vi "Init.vi"(8 "error in (no error)":errorcluster, 11 "RT_Sprite in":refnum<class "RT_Sprite.lvclass">) -> (0 "error out":errorcluster, 3 "RT_Sprite out":refnum<class "RT_Sprite.lvclass">)   [LabVIEW 2019, in "RT_Game.lvlib" / "RT_Sprite.lvclass"]
uses:
  RT_Sprite.lvclass
  GameObject/GameObject.lvclass
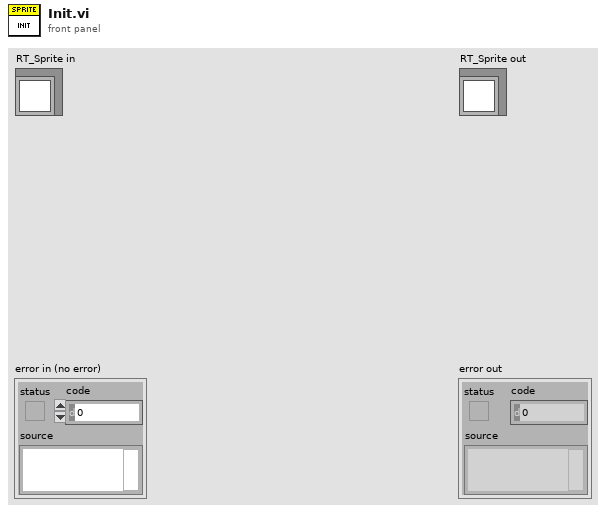
[diagram p1: front panel]
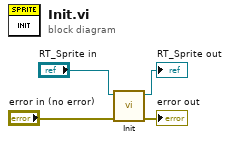
[diagram p0: block diagram]
diagram:
  n1 = call-parent "Init.vi"("error in (no error)"="error in (no error)", "GameObject in"="RT_Sprite in") -> ("error out"=→"error out":errorcluster, "GameObject out"=→"RT_Sprite out":refnum<class "RT_Sprite.lvclass">)  [unwired: 8 in]
